vi "NI VeriStand - Set Custom Device Decimation.vi"(8 "error in (no error)":errorcluster, 10 "Decimation":i32, 11 "Device Ref in":T1 format="%.0x") -> (0 "error out":errorcluster, 3 "Device Ref out":T1 format="%.0x")   [LabVIEW 2026, in "Custom Devices Storage.lvlib"]
uses:
  Custom Devices Storage.lvlib
  <vilib>/NI VeriStand/Custom Device API/Custom Device Item Ref.ctl
  C:/Users/Administrator/Desktop/Jatin/All DNC DLLs/NationalInstruments.VeriStand.SystemDefinitionAPI.dll
  Jatin/All DNC DLLs/NationalInstruments.VeriStand.SystemDefinitionAPI.dll
  <vilib>/NI VeriStand/Custom Device API/Custom Device API.lvlib
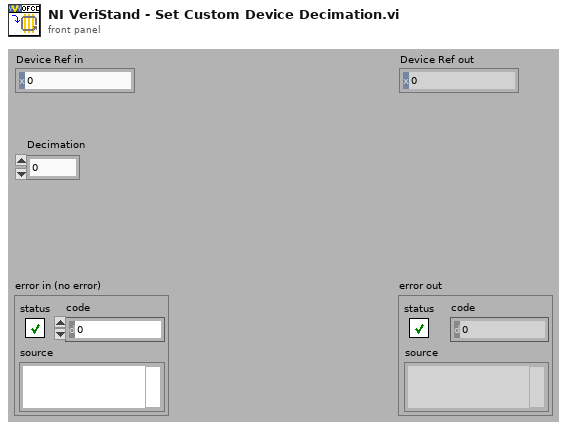
[diagram p1: front panel]
types:
  T1 = typedef "Custom Device API.lvlib/Custom Device Item Ref.ctl" = u64
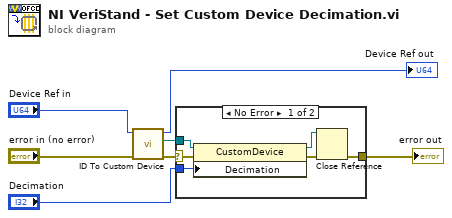
[diagram p0: block diagram]
diagram:
  n1 = call "ID To Custom Device.vi"("error in (no error)"="error in (no error)", "ID in"="Device Ref in") -> ("error out"=w5:errorcluster, "NationalInstruments.VeriStand.SystemDefinitionAPI.CustomDevice"=w3:refnum<k39>, "ID out"=→"Device Ref out":u64)  [unwired: 7 in]
  n2 = case shown="No Error" w5 {
    selector: w5 -> [w13 w14]
    tunnel: w3 -> [w12 _]
    tunnel: "Decimation" -> [w11 _]
    tunnel: [w8 w14] -> w1
    frame No Error {
      n3 = property class="CustomDevice"(reference=w12, error in=w13, "Decimation"=w11) -> (reference out=w9:refnum<k39>, error out=w10:errorcluster)
      n4 = Close Reference(reference=w9, error in (no error)=w10) -> (error out=w8:errorcluster)
    }
    frame Error {
    }
  }
  "error out" <- w1
